vi "xss-ypi-control.vi"(5 "Ki-xy":sgl=0.001 format="%#_13g", 8 "xy-ref":fxp<+/-,18,5>[](array[numeric])=[0.0, 0.0], 9 "ControlParamsLin":T1={"umax"=3.0, "Ns_obs/cntrl"=0, "ref_f_VEC"=[0.0, 0.0], "du_max"=0.0, "Nbar"=0.0}, 11 "x_k-y_k":fxp<+/-,25,6>[](array[numeric])=[0.0, 0.0]) -> (0 "u_y saturated":bool, 1 "u_x saturated":bool, 2 "sat(u_y)":fxp<+/-,18,5>, 3 "u_k (saturated)":fxp<+/-,32,5>)   [LabVIEW 2017]
uses:
  fpga_subVIs_ssxy/fixed-point-ss/typeDefs/FXPControlParams_distEst.ctl
panel:
  out "sat(u_x)":fxp<+/-,18,5>
  out "del u(k)":fxp<+/-,64,15>
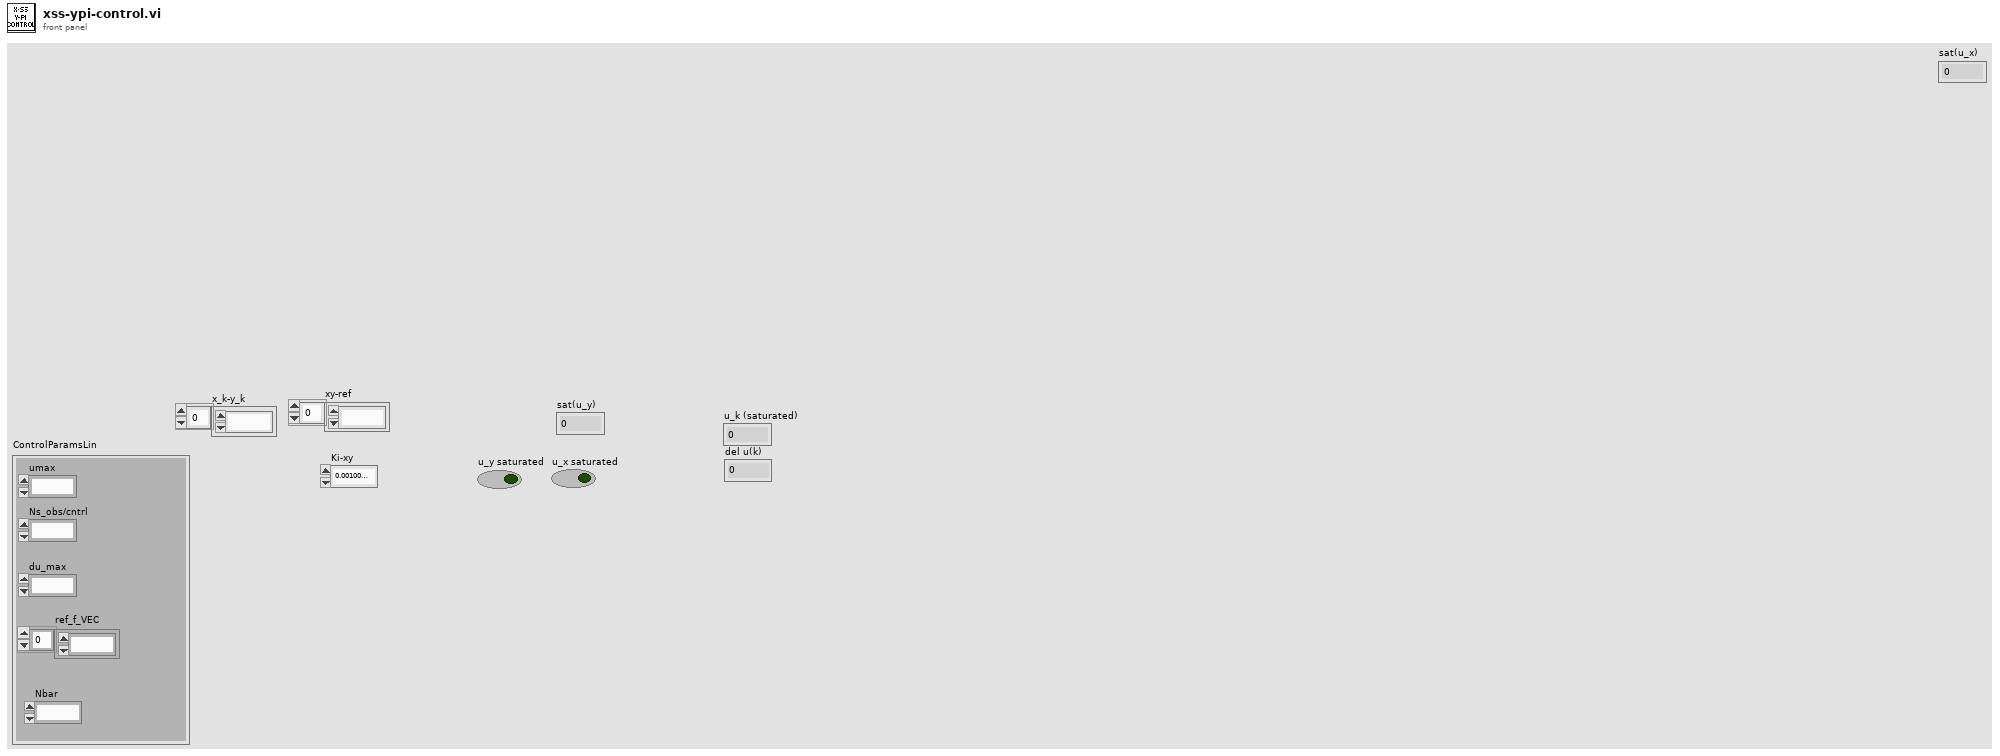
[diagram p1: front panel]
types:
  T1 = typedef "FXPControlParams_distEst.ctl" = cluster{"umax":fxp<+/-,18,5>, "Ns_obs/cntrl":u8, "ref_f_VEC":fxp<+/-,32,5>[], "du_max":fxp<+/-,18,5>, "Nbar":fxp<+/-,32,5>}
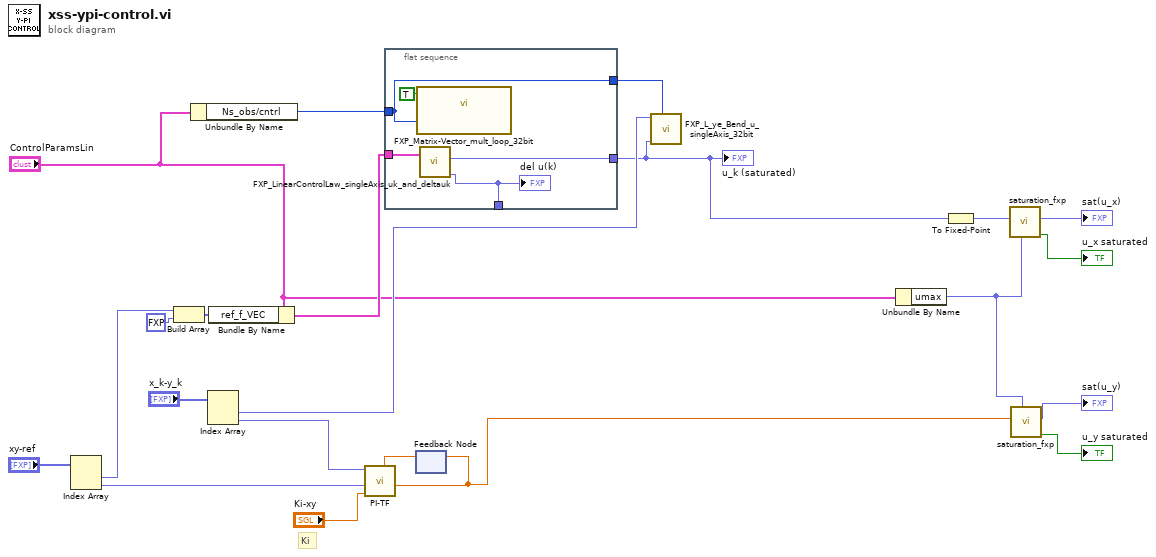
[diagram p0: block diagram]
diagram:
  # "Ki"
  n1 = Index Array(array="xy-ref") -> (element #1=w14:fxp<+/-,18,5>, element #2=w19:fxp<+/-,18,5>)  [unwired: 2 in]
  n2 = Build Array(w14, fxp<+,1,1> 0.0) -> (w16:fxp<+/-,18,5>[])
  n3 = Unbundle By Name("ControlParamsLin") -> ("Ns_obs/cntrl"=w1:u8)
  n4 = Index Array(array="x_k-y_k") -> (element #1=w12:fxp<+/-,25,6>, element #2=w17:fxp<+/-,25,6>)  [unwired: 2 in]
  n5 = Bundle By Name(cluster="ControlParamsLin", "ref_f_VEC"=w16) -> (w13:T1)
  n6 = flat-sequence {
    tunnel: w1 -> [w25]
    tunnel: w13 -> [w27]
    tunnel: [w26] -> _
    tunnel: [w25] -> w11
    tunnel: [w24] -> w9
    frame #0 {
      n7 = call "FXP_Matrix-Vector_mult_loop_32bit.vi"("Ns_1"=w25, "inputValid"=TRUE) -> ()  [unwired: 9 in, 1 out]
      n8 = call "FXP_LinearControlLaw_singleAxis_uk_and_deltauk.vi"("ControlParams_distEst"=w27) -> ("del u_x"=w26:fxp<+/-,64,15>, "u_k (un saturated)"=w24:fxp<+/-,32,5>)  [unwired: 9 in]
      "del u(k)" <- w26
    }
  }
  n9 = feedback #1() -> (w22:sgl)  [unwired: 1 in]
  n10 = call "PI-TF.vi"("u(k-1)"=w22, "Ki"="Ki-xy", "setpoint"=w19, "y(k)"=w17) -> ("u(k)"=w4:sgl)  [unwired: 7 in]
  n11 = feedback-in #1(w4) -> ()
  n12 = call "FXP_L_ye_Bend_u_singleAxis_32bit.vi"("NS"=w11, "U(k): ux"=w9, "Y(k): x"=w12) -> ()  [unwired: 7 in, 2 out]
  n13 = Unbundle By Name("ControlParamsLin") -> ("umax"=w3:fxp<+/-,18,5>)
  n14 = To Fixed-Point(number=w9) -> (fixed-point=w10:fxp<+/-,32,5>)  [unwired: 1 in]
  n15 = call "saturation_fxp.vi"("uMax"=w3, "signal_in"=w10) -> ("has_saturated"=→"u_x saturated":bool, "signal_out (saturated)"=→"sat(u_x)":fxp<+/-,18,5>)  [unwired: 8 in]
  n16 = call "saturation_fxp.vi"("uMax"=w3, "signal_in"=w4) -> ("has_saturated"=→"u_y saturated":bool, "signal_out (saturated)"=→"sat(u_y)":fxp<+/-,18,5>)  [unwired: 8 in]
  "u_k (saturated)" <- w9
